vi "readnoerror.vi"(10 "error in (no error)":errorcluster, 11 "Slave Address (7-bit)":u8 format="%x") -> (0 "error out":errorcluster, 2 "Reading":dbl)   [LabVIEW 2015]
uses:
  <vilib>/myRIO/Instrument Drivers/Onboard IO/I2C/typedefs/I2C User Configuration.ctl
  <vilib>/myRIO/Instrument Drivers/Onboard IO/I2C/typedefs/I2C Transfer Rate.ctl
  <vilib>/myRIO/Instrument Drivers/Onboard IO/I2C/typedefs/I2C Reference.ctl
  <vilib>/myRIO/Common/Instrument Driver Framework/Utilities/typedefs/myRIO Generic Hardware Reference.ctl
  <vilib>/myRIO/Common/Instrument Driver Framework/Utilities/typedefs/Hardware Version Enum.ctl
  <vilib>/myRIO/Common/Instrument Driver Framework/Utilities/typedefs/myRIO v1.0 Reference.ctl
  <vilib>/myRIO/Common/Instrument Driver Framework/Utilities/typedefs/Generic FPGA Reference.ctl
  <vilib>/myRIO/Common/Instrument Driver Framework/myRIO v1.0/I2C/typedefs/I2C Channels Enum.ctl
  <vilib>/myRIO/Instrument Drivers/Onboard IO/I2C/typedefs/I2C Configuration.ctl
  <vilib>/userdefined/High Color/nirio_resource_hc.ctl
  <vilib>/myRIO/Common/Instrument Driver Framework/Utilities/vis/Is FPGA Ref Available.vi
  <vilib>/myRIO/Common/Instrument Driver Framework/myRIO v1.0/I2C/vis/myRIO v1.1 Open I2C.vi
  <vilib>/myRIO/Instrument Drivers/Onboard IO/I2C/vis/Configure.vi
  <vilib>/myRIO/Instrument Drivers/Onboard IO/I2C/vis/Write.vi
  <vilib>/myRIO/Instrument Drivers/Onboard IO/I2C/vis/Read.vi
  <vilib>/myRIO/Common/Instrument Driver Framework/Utilities/vis/Validate Channels.vi
  <vilib>/myRIO/Common/Instrument Driver Framework/myRIO v1.0/I2C/vis/myRIO v1.0 Reserve I2C.vi
  <vilib>/myRIO/Common/Instrument Driver Framework/myRIO v1.0/I2C/vis/myRIO v1.0 Build MUX Configuration I2C.vi
  <vilib>/myRIO/Common/Instrument Driver Framework/myRIO v1.0/Resource Manager/vis/myRIO v1.0 Reserve Channel List.vi
  <vilib>/myRIO/Common/Instrument Driver Framework/myRIO v1.0/Resource Manager/vis/myRIO v1.0 Create Configuration List.vi
  <vilib>/myRIO/Common/Instrument Driver Framework/myRIO v1.0/Resource Manager/vis/myRIO v1.0 Reserve Channel.vi
  <vilib>/myRIO/Common/Instrument Driver Framework/myRIO v1.0/Resource Manager/vis/myRIO v1.0 Unreserve Channel.vi
  <vilib>/myRIO/Common/Instrument Driver Framework/myRIO v1.0/Resource Manager/vis/myRIO v1.0 Build Mutex Name.vi
  <vilib>/Utility/VariantDataType/GetNumericInfo.vi
  <vilib>/Utility/error.llb/Error Cluster From Error Code.vi
  <vilib>/myRIO/Common/Instrument Driver Framework/myRIO v1.0/myRIO v1.1 Open.vi
  <vilib>/myRIO/Common/Instrument Driver Framework/Utilities/vis/IO Manager.vi
  <vilib>/myRIO/Common/Instrument Driver Framework/Utilities/vis/Configuration Manager.vi
  <vilib>/myRIO/Common/Instrument Driver Framework/myRIO v1.0/Resource Manager/vis/myRIO v1.0 Configure IO.vi
  <vilib>/myRIO/Common/Instrument Driver Framework/myRIO v1.0/myRIO v1.0 Close.vi
  <vilib>/myRIO/Common/Instrument Driver Framework/myRIO v1.0/I2C/vis/myRIO v1.0 Configure I2C.vi
  <vilib>/myRIO/Common/Instrument Driver Framework/myRIO v1.0/I2C/vis/myRIO v1.0 Write I2C.vi
  <vilib>/myRIO/Common/Instrument Driver Framework/myRIO v1.0/I2C/vis/myRIO v1.0 Read I2C.vi
  <vilib>/myRIO/Express VI/Onboard IO/I2C/I2C Express VI.xnode
  <vilib>/myRIO/Instrument Drivers/Onboard IO/I2C/vis/myRIO I2C Open.xnode
  <vilib>/myRIO/Instrument Drivers/Onboard IO/I2C/I2C.lvlib
panel:
  out "x":dbl
  in  "Differences":dbl[](array[numeric])
  in  "Three readings":dbl[](array[numeric])
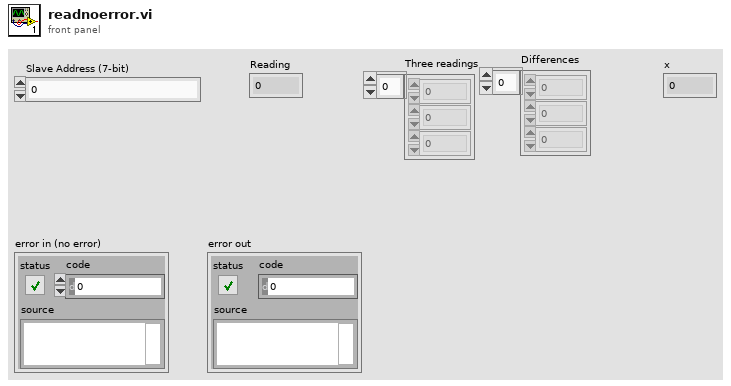
[diagram p1: front panel]
types:
  T1 = typedef "I2C.lvlib/I2C Reference.ctl" = cluster{"myRIO Reference":T2, "I2C Channels Enum":T6, "I2C Configuration":T7}
  T2 = typedef "myRIO Generic Hardware Reference.ctl" = cluster{"myRIO Model":T3, "myRIO Hardware Reference":T4}
  T3 = typedef "Hardware Version Enum.ctl" = enum16{"Unknown", "myRIO-1900", "myRIO-1950", "roboRIO"}
  T4 = typedef "myRIO v1.0 Reference.ctl" = cluster{"Generic FPGA Reference":T5, "Allow multiple opens":bool}
  T5 = typedef "Generic FPGA Reference.ctl" = refnum<k20>
  T6 = typedef "I2C Channels Enum.ctl" = enum16{"Not Connected", "A/I2C", "B/I2C", "I2C/I2C"}
  T7 = typedef "I2C.lvlib/I2C Configuration.ctl" = cluster{"I2C Transfer Rate":T8}
  T8 = typedef "I2C.lvlib/I2C Transfer Rate.ctl" = enum16{"Standard mode (100 kbps)", "Fast mode (400 kbps)"}
  T9 = typedef "I2C.lvlib/I2C User Configuration.ctl" = cluster{"I2C Transfer Rate":T8}
  T10 = typedef "nirio_resource_hc.ctl" = tag
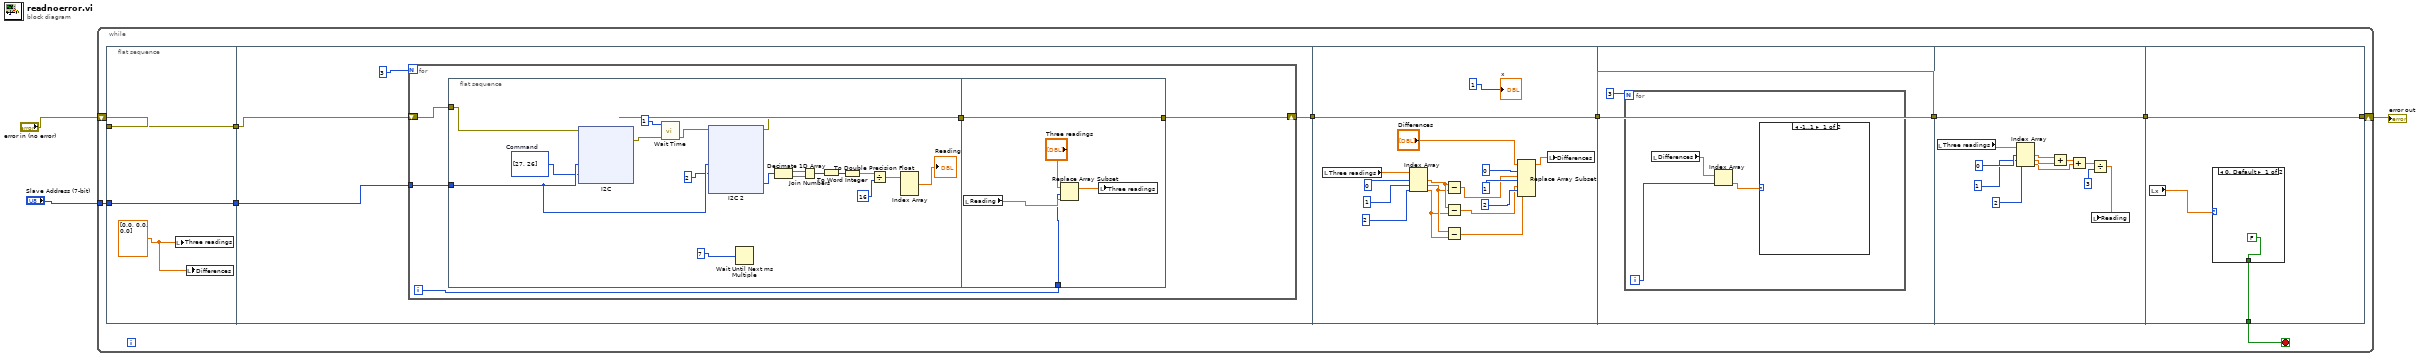
[diagram p0: block diagram]
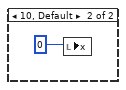
[diagram p2: hidden frame]
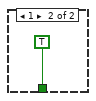
[diagram p3: hidden frame]
diagram:
  n1 = while {
    tunnel: "Slave Address (7-bit)" -> [w9]
    shift-right: [w10] -> w3
    shift-left: "error in (no error)" -> [w8]
    stop <- w7 stop-if-true
    n2 = flat-sequence {
      tunnel: w8 -> [w15]
      tunnel: w9 -> [w16]
      tunnel: [w16] -> w5
      tunnel: [w15] -> w4
      tunnel: [w20] -> w6
      tunnel: w5 -> [w19]
      tunnel: w4 -> [w18]
      tunnel: w6 -> [w142]
      tunnel: [w142] -> w13
      tunnel: w13 -> [w144]
      tunnel: [w144] -> w12
      tunnel: w12 -> [w160]
      tunnel: [w160] -> w11
      tunnel: [w163] -> w10
      tunnel: w11 -> [w163]
      tunnel: [w161] -> w7
      frame #0 {
        w14 = dbl[] [0.0, 0.0, 0.0]
        n3 = local write "Three readings"(w14) -> ()
        n4 = local write "Differences"(w14) -> ()
      }
      frame #1 {
        n5 = for {
          N: 3 -> [_]
          tunnel: w19 -> [w24]
          shift-right: [w25] -> w20
          shift-left: w18 -> [w23]
          i -> [w22]
          n6 = flat-sequence {
            tunnel: w24 -> [w42]
            tunnel: w23 -> [w39]
            tunnel: [w36] -> w21
            tunnel: [w125] -> w25
            tunnel: w21 -> [w125]
            tunnel: w22 -> [w121]
            frame #0 {
              w40 = u8[] [27, 26]  # Command
              n7 = xnode "I2C"("Slave Address (7-bit)"=w42, "Bytes to Write"=w40, "error in (no error)"=w39) -> ("error out"=w38:errorcluster)
              n8 = call "Wait Time.vi"("error in (no error)"=w38, "Wait Time (ms)"=1) -> ("error out"=w37:errorcluster)  [unwired: 9 in]
              n9 = xnode "I2C 2"("Slave Address (7-bit)"=w42, "Byte Count"=2, "error in (no error)"=w37) -> ("Bytes Read"=w26:u8[], "error out"=w36:errorcluster)
              n10 = Wait Until Next ms Multiple(millisecond multiple=7) -> ()  [unwired: 1 out]
              n11 = Decimate 1D Array(w26) -> (w33:u8[], w34:u8[])
              n12 = Join Numbers(hi=w33, lo=w34) -> ((hi.lo)=w32:u16[])
              n13 = To Word Integer(number=w32) -> (16bit integer=w31:i16[])
              n14 = To Double Precision Float(number=w31) -> (double precision float=w30:dbl[])
              n15 = Divide(x=w30, y=16) -> (x/y=w29:dbl[])
              n16 = Index Array(array=w29) -> (element #1=→"Reading":dbl)  [unwired: 3 in, 2 out]
            }
            frame #1 {
              n17 = local read "Reading"() -> (w124:dbl)
              n18 = Replace Array Subset(array="Three readings", new element=w124, index=w121) -> (w123:dbl[])
              n19 = local write "Three readings"(w123) -> ()
            }
          }
        }
      }
      frame #2 {
        n20 = local read "Three readings"() -> (w141:dbl[])
        n21 = Index Array(array=w141, index #1=0, index #2=1, index #3=2) -> (element #1=w135:dbl, element #2=w134:dbl, element #3=w133:dbl)
        n22 = Subtract(x=w135, y=w134) -> (x-y=w132:dbl)
        n23 = Subtract(x=w135, y=w133) -> (x-y=w130:dbl)
        n24 = Subtract(x=w134, y=w133) -> (x-y=w129:dbl)
        n25 = Replace Array Subset(array="Differences", new element #1=w132, index #1=0, new element #2=w130, index #2=1, new element #3=w129, index #3=2) -> (w127:dbl[])
        n26 = local write "Differences"(w127) -> ()
        "x" <- 1
      }
      frame #3 {
        n27 = for {
          N: 3 -> [_]
          i -> [w147]
          n28 = local read "Differences"() -> (w146:dbl[])
          n29 = Index Array(array=w146, index=w147) -> (element=w145:dbl)
          n30 = case shown="-1..1" w145 {
            frame -1..1 {
            }
            frame 10, Default {
              n31 = local write "x"(0) -> ()
            }
          }
        }
      }
      frame #4 {
        n32 = local read "Three readings"() -> (w159:dbl[])
        n33 = Index Array(array=w159, index #1=0, index #2=1, index #3=2) -> (element #1=w158:dbl, element #2=w157:dbl, element #3=w155:dbl)
        n34 = Add(x=w158, y=w157) -> (x+y=w156:dbl)
        n35 = Add(x=w156, y=w155) -> (x+y=w154:dbl)
        n36 = Divide(x=w154, y=3) -> (x/y=w152:dbl)
        n37 = local write "Reading"(w152) -> ()
      }
      frame #5 {
        n38 = local read "x"() -> (w162:dbl)
        n39 = case shown="0, Default" w162 {
          tunnel: [FALSE TRUE] -> w161
          frame 0, Default {
          }
          frame 1 {
          }
        }
      }
    }
  }
  "error out" <- w3
